vi "CHD_SIM_SIM_MODULE_INIT.vi"(3 "Module Index":i32, 5 "Drive PWM Channel":T2, 6 "DriveDistPerCount":dbl=1.0, 10 "Drive B Channel":T1, 11 "Drive A channel":T1) -> ()   [LabVIEW 2019]
uses:
  <vilib>/Rock Robotics/SystemInterfaces/DIO/FPGA_DIOPWMChannel.ctl
  <vilib>/Rock Robotics/SystemInterfaces/DIO/FPGA_DIOChannel.ctl
  CHD_SIM_SIM_Globals.vi
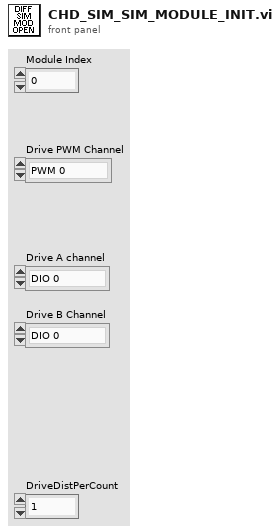
[diagram p1: front panel]
types:
  T1 = typedef "FPGA_DIOChannel.ctl" = enum8{"DIO 0", "DIO 1", "DIO 2", "DIO 3", "DIO 4", "DIO 5", "DIO 6", "DIO 7", "DIO 8", "DIO 9", "DIO MXP 0", "DIO MXP 1", "DIO MXP 2", "DIO MXP 3", "DIO MXP 4", "DIO MXP 5", "DIO MXP 6", "DIO MXP 7", "DIO MXP 8", "DIO MXP 9", "DIO MXP 10", "DIO MXP 11", "DIO MXP 12", "DIO MXP 13", "DIO MXP 14", "DIO MXP 15", "SPI Port CS1", "SPI Port CS2", "SPI Port CS3", "SPI Port MISO", "SPI Port MOSI", "Invalid"}
  T2 = typedef "FPGA_DIOPWMChannel.ctl" = enum8{"PWM 0", "PWM 1", "PWM 2", "PWM 3", "PWM 4", "PWM 5", "PWM 6", "PWM 7", "PWM 8", "PWM 9", "PWM MXP 0", "PWM MXP 1", "PWM MXP 2", "PWM MXP 3", "PWM MXP 4", "PWM MXP 5", "PWM MXP 6", "PWM MXP 7", "PWM MXP 8", "PWM MXP 9", "Invalid"}
  T3 = cluster{"Drive Motor Device Index":i32, "Drive Encoder Device Index":i32, "Drive DistPerzcount":dbl}[]
  T4 = typedef "CHD_DRIVE_MODULE_TYPDEF.ctl" = cluster{"DiffDriveMotor":T5, "DiffDriveEnc":T8}
  T5 = typedef "WPI_MotorControlDeviceRef.ctl" = cluster{"DeviceStatus":errorcluster, "Type":T6, "PWM":cluster{"PWM Channel":T2, "DeadBand":T7}, "CAN":cluster{"Device Number":u8, "SetOutput VI Ref":variant, "GetOutput VI Ref":variant, "Enable VI Ref":variant, "Disable VI Ref":variant, "Data":variant}, "Invert":bool, "DIO PWM":cluster{"PWM \"Enable\" Channel":T2, "DIOChannel":T1, "PWM Rate":dbl}}
  T6 = typedef "WPI_MotorControlType.ctl" = enum16{"PWM", "CAN", "DIO PWM"}
  T7 = typedef "WPI_PWMDeadband.ctl" = cluster{"Name":string, "maxPositivePwm":i32, "minPositivePwm":i32, "centerPwm":i32, "maxNegativePwm":i32, "minNegativePwm":i32, "angularRange":u16}
  T8 = typedef "WPI_EncoderDevRef.ctl" = cluster{"DevStatus":errorcluster, "EncoderIndex":T9, "CounterIndex":T10, "DistancePerCount":dbl, "Decoding Type":T11}
  T9 = typedef "FPGA_EncoderIdx.ctl" = enum8{"Enc 0", "Enc 1", "Enc 2", "Enc 3", "Enc 4", "Enc 5", "Enc 6", "Enc 7", "Invalid"}
  T10 = typedef "FPGA_CounterCtrSystemIndex.ctl" = enum8{"Ctr 0", "Ctr 1", "Ctr 2", "Ctr 3", "Ctr 4", "Ctr 5", "Ctr 6", "Ctr 7", "Invalid"}
  T11 = typedef "WPI_EncoderType.ctl" = enum16{"1x", "2x", "4x"}
  T12 = cluster{"Drive Motor Device Index":i32, "Drive Encoder Device Index":i32, "Drive DistPerzcount":dbl}
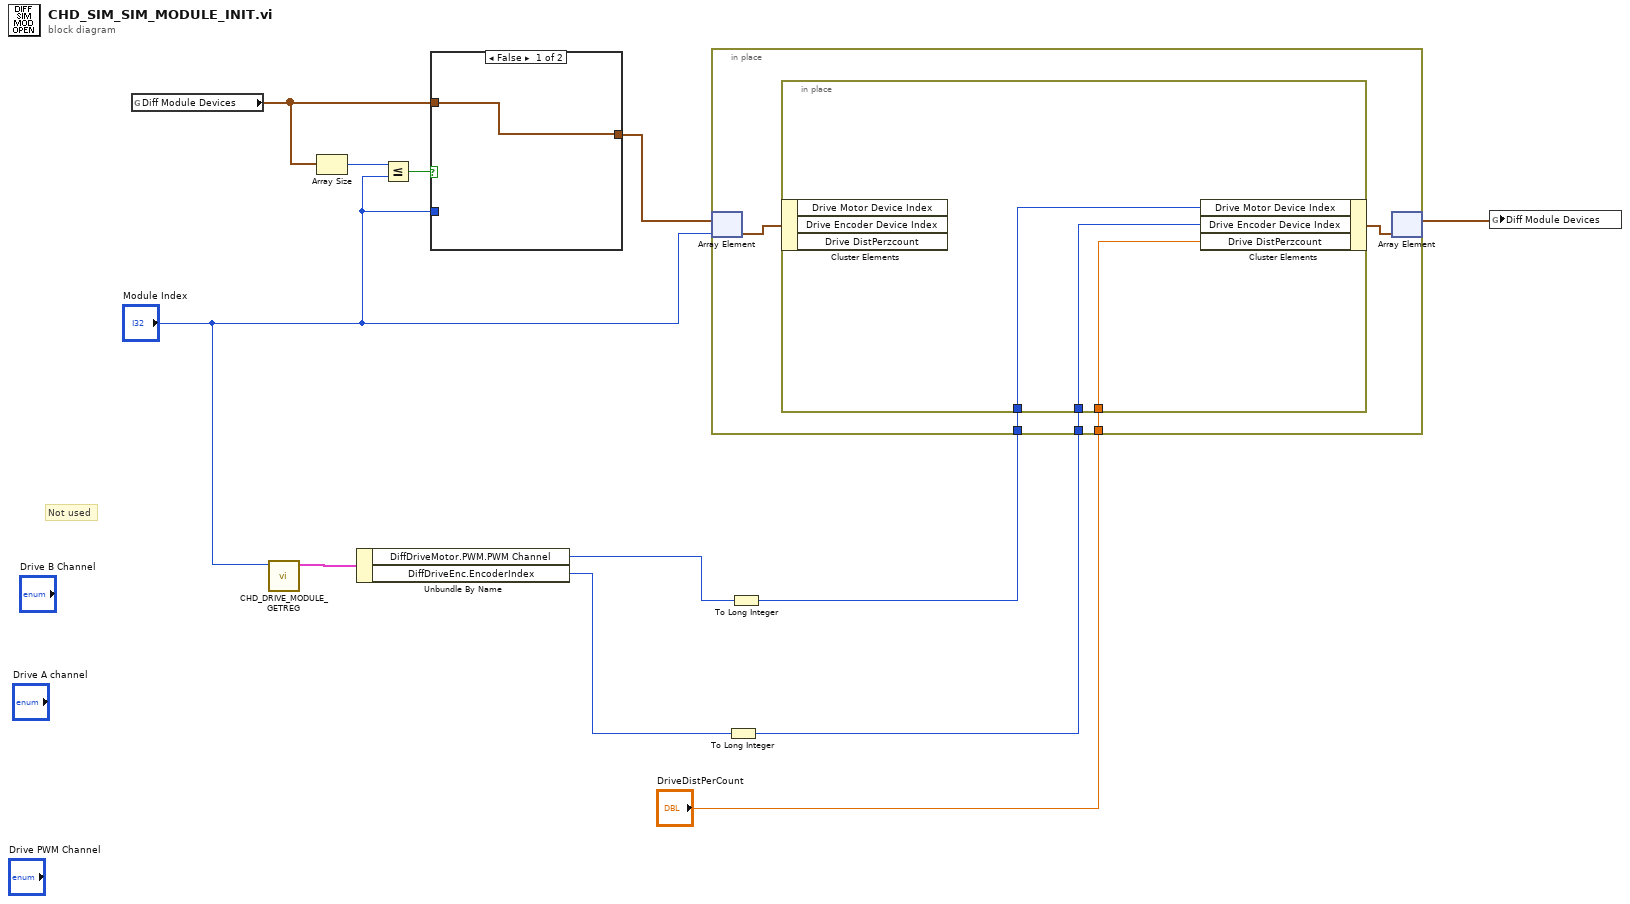
[diagram p0: block diagram]
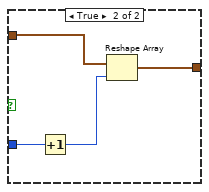
[diagram p2: hidden frame]
diagram:
  # "Not used"
  n1 = global read "CHD_SIM_SIM_Globals.vi" "Diff Module Devices"() -> (w6:T3)
  n2 = call "CHD_DRIVE_MODULE_GETREG.vi"("Suffix"="Module Index") -> ("Diff Module TypDef"=w4:T4)  [unwired: 10 in]
  n3 = Array Size(array=w6) -> (size(s)=w8:i32)
  n4 = Unbundle By Name(w4) -> ("DiffDriveMotor.PWM.PWM Channel"=w1:T2, "DiffDriveEnc.EncoderIndex"=w2:T9)
  n5 = Less Or Equal?(x=w8, y="Module Index") -> (x <= y?=w7:bool)
  n6 = case shown="False" w7 {
    tunnel: w6 -> [w13 w15]
    tunnel: "Module Index" -> [_ w17]
    tunnel: [w13 w14] -> w5
    frame False {
    }
    frame True {
      n7 = Increment(x=w17) -> (x+1=w16:i32)
      n8 = Reshape Array(w15, w16) -> (w14:T3)
    }
  }
  n9 = To Long Integer(number=w2) -> (32bit integer=w10:i32)
  n10 = To Long Integer(number=w1) -> (32bit integer=w11:i32)
  n11 = in-place {
    in-place-border: w11 -> [w21]
    in-place-border: w10 -> [w19]
    in-place-border: "DriveDistPerCount" -> [w18]
    n12 = in-place-array #1(w5, "Module Index") -> (w22:T12)
    n13 = in-place {
      in-place-border: w21 -> [w25]
      in-place-border: w19 -> [w24]
      in-place-border: w18 -> [w23]
      n14 = in-place-cluster #2(w22) -> ()  [unwired: 3 out]
      n15 = in-place-cluster #2("Drive Motor Device Index"=w25, "Drive Encoder Device Index"=w24, "Drive DistPerzcount"=w23) -> (w20:T12)
    }
    n16 = in-place-array #1(w20) -> (w12:T3)  [unwired: 1 out]
  }
  n17 = global write "CHD_SIM_SIM_Globals.vi" "Diff Module Devices"(w12) -> ()
